vi "GUI.vi"() -> ()   [LabVIEW 2018]
uses:
  <vilib>/robotics/Kinematics/NI_Kinematics.lvlib
  <vilib>/robotics/Kinematics/Analytical/NI_Robotics_AnalyticKinematics.lvlib
  <vilib>/robotics/Kinematics/Robot/Inverse Kinematics (Point).vi
  <vilib>/robotics/Kinematics/Analytical/SCARA/SCARA Inverse Kinematics.vi
  <vilib>/robotics/Kinematics/Analytical/SCARA/NI_Robotics_SCARA Serial Arm Class.lvclass
panel:
  out "Power 2":bool
  out "Angle 6":dbl
  out "Angle 5":dbl
  out "Angle 4":dbl
  out "Angle 3":dbl
  out "Angle 2":dbl
  out "Angle 1":dbl
  out "Image":T1(plugin-control)
  out "Apples Grabbed":dbl
  in  "Stop":bool
  in  "Start":bool
  in  "Home":bool
  in  "Power":bool
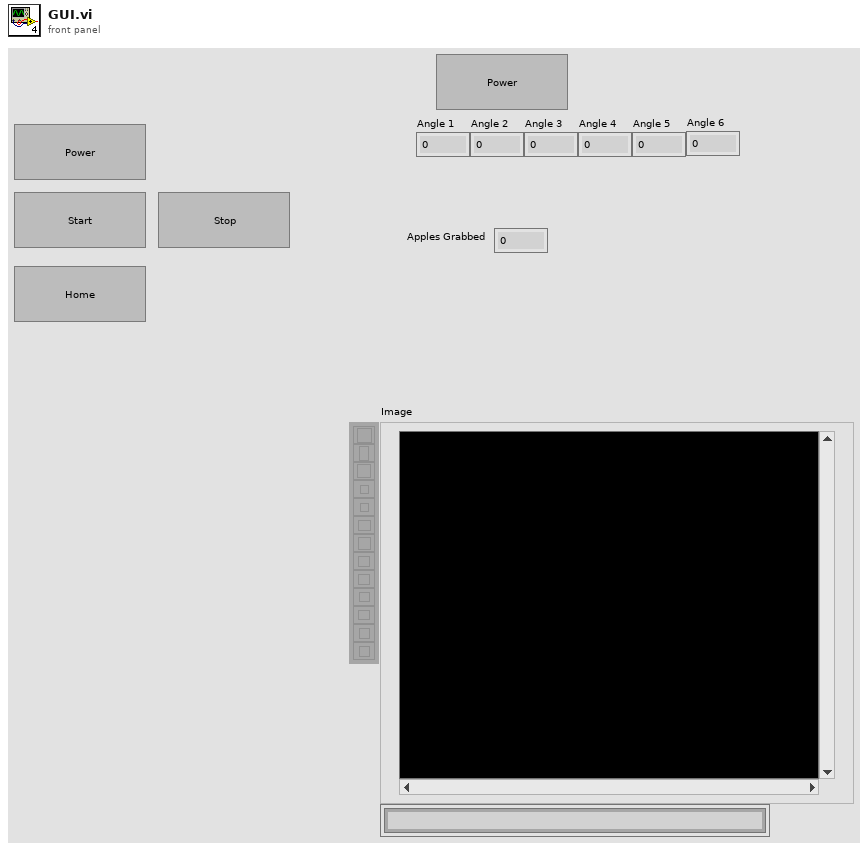
[diagram p1: front panel]
types:
  T1 = typedef "IMAQ Image.ctl" = refnum<image>
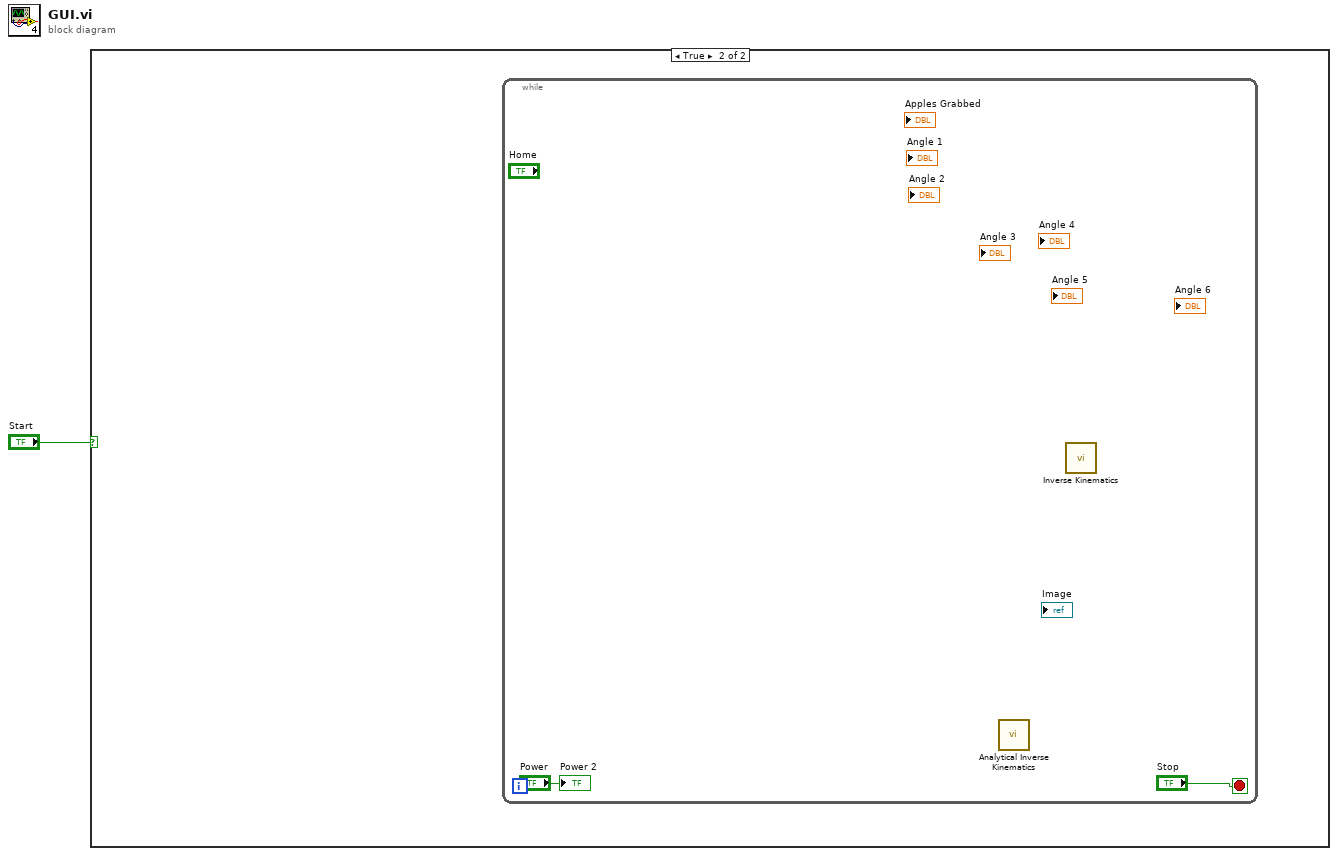
[diagram p0: block diagram]
diagram:
  n1 = case shown="True" "Start" {
    frame False {
    }
    frame True {
      n2 = while {
        stop <- "Stop" stop-if-true
        n3 = call-poly <vilib>:"Analytical Inverse Kinematics.vi"() -> ()  [unwired: 9 in, 3 out]
        n4 = call-poly <vilib>:"Inverse Kinematics.vi"() -> ()  [unwired: 8 in, 4 out]
        "Power 2" <- "Power"
      }
    }
  }
